vi "RT Driver VI.vi"(6 "Device Clock":string, 9 "Device Inputs FIFO":refnum<k33>, 10 "Device Outputs FIFO":refnum<k33>, 11 "Device Reference":T1 format="%.0x") -> ()   [LabVIEW 2020, in "Waveform Analog Output Engine.lvlib"]
uses:
  Waveform Analog Output Engine.lvlib
  <vilib>/NI VeriStand/Custom Device API/Custom Device Item Ref.ctl
  <vilib>/NI VeriStand/Custom Device API/Custom Device Channel Type.ctl
  <vilib>/Platform/TimedLoop/XDataNode/timing_clust.ctl
  <vilib>/Platform/TimedLoop/XDataNode/nitl_modes.ctl
  <vilib>/Platform/TimedLoop/XDataNode/wakeup.ctl
  <vilib>/NI VeriStand/Custom Device API/Message Response (String).ctl
  <vilib>/NI VeriStand/Custom Device API/Message Response (Byte Array).ctl
  <vilib>/DAQmx/write.llb/DAQmx Write (Analog 1D Wfm NChan NSamp).vi
  <vilib>/DAQmx/miscellaneous.llb/DAQmx Fill In Error Info.vi
  <vilib>/platform/TimedLoop/XDataNode/XDataNode.xnode
  <vilib>/NI VeriStand/Custom Device API/Custom Device API.lvlib
  <vilib>/NI VeriStand/Custom Device Tools/Custom Device Utility Library/Custom Device Utility Library.lvlib
  <resource>/objmgr/daqmx.rc
  <vilib>/Platform/TimedLoop/XDataNode/XDNodeRunTimeDep.lvlib
panel:
  out "Number of Overflow Occurred":i32
  out "Number of Underflow Occurred":i32
  out "L2 Output Buffer Usage":i32
  out "Actual Update Interval_Data Loop":dbl
  out "DAQ Error Code":i32
  out "Actual Update Interval_DAQ Loop":dbl
  out "Actual Sample Rate":dbl
  in  "Initialization Status Notifier":refnum<notifier>
  in  "Status Notifier":refnum<notifier>
  # "Custom Device Template\nv1.0"
  # "Use this template as a starting point for creating a custom device code module. The input controls shown here are specially named controls that the system will use to provide the device loop with data. The controls are not required for the device loop to run. For instance, if the device doesn't produce any output data, then you don't need the Device Outputs FIFO control. If you do use these controls, however, they need to have these exact names to be functional."
  # "status chs"
  # "The optional status notifier element is used to notify the RT engine of the last state of the custom device, and to indicate the device has completed execution. If this control is not used, a default No Error value is returned to the system when the device finishes execution.\n\nNote: This error state is not checked until the system shuts down. Use an output status channel to send more immediate status values to the system."
  # "This optional input can be used to send the VeriStand Engine the final status of the custom device initalization process. If this control exists on the custom device front panel, the VeriStand Engine will wait for a status update before starting up. If the custom device reports an error, that will abort the execution of the current configuration in the VeriStand Engine.\n\nThis control can be deleted if the custom device does not need to send the initialization status update."
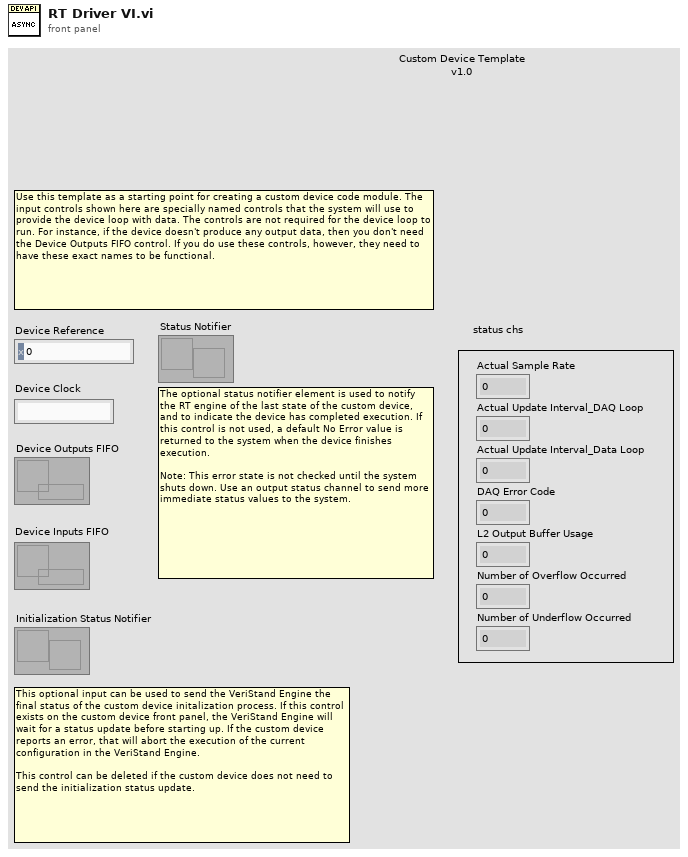
[diagram p1: front panel]
types:
  T1 = typedef "Custom Device API.lvlib/Custom Device Item Ref.ctl" = u64
  T2 = typedef "Custom Device API.lvlib/Custom Device Channel Type.ctl" = enum16{"Input", "Output"}
  T3 = typedef "Custom Device API.lvlib/Custom Device Engine Event Ref.ctl" = refnum<event-registration>
  T4 = typedef "Custom Device API.lvlib/Custom Device Timed Loop Priority.ctl" = enum32{"Low", "Medium", "High"}
  T5 = typedef "XDNodeRunTimeDep.lvlib/timing_clust.ctl" = cluster{"Expected End [f-1]":u64, "Actual End [f-1]":u64, "Finished Late? [f-1]":bool, "Expected End [i-1]":u64, "Actual End [i-1]":u64, "Finished Late? [i-1]":bool, "Expected Start [i]":u64, "Actual Start [i]":u64, "Expected Start [f]":u64, "Actual Start [f]":u64, "Source Name":string, "Structure Name":string, "Period":i64, "Deadline":i64, "Offset":i64, "Start":i64, "Priority":i32, "Timeout":i32, "Mode":T6, "Wakeup Reason":T7, "Error":errorcluster, "Source Type":string, "Secondary Source Type":string, "Global End Time":u64, "Global Start Time":u64, "Frame Duration":u64, "Iteration Duration":u64, "Assigned CPU":i32, "I/O Scan Engine Mode":u32}
  T6 = typedef "XDNodeRunTimeDep.lvlib/nitl_modes.ctl" = enum32{"No Change", "Process missed periods, maintain original phase", "Discard missed periods, maintain original phase", "Process missed periods, ignore original phase", "Discard missed periods, ignore original phase"}
  T7 = typedef "XDNodeRunTimeDep.lvlib/wakeup.ctl" = enum32{"Normal", "Aborted", "Asynchronous wakeup", "Timing source error", "Timed loop error", "Timeout"}
  T8 = typedef "Custom Device API.lvlib/Message Response (String).ctl" = cluster{"Response":string, "Error":errorcluster}
  T9 = typedef "Custom Device API.lvlib/Message Response (Byte Array).ctl" = cluster{"Response":u8[], "Error":errorcluster}
  T10 = typedef "Waveform Analog Output Engine.lvlib/DAQ Config Data.ctl" = cluster{"DAQPhysicalChannel(s)":string, "SampleRate":dbl, "MaxV":dbl, "MinV":dbl, "#Samples":dbl, "DataLoopInterval(ms)":u32, "StartDelay(ms)":dbl, "#L1OutputBuffers":i32, "#L2OutputBuffers":i32, "#Channels":i32, "ActualSampleRate(Hz)":dbl, "DAQTaskRef":refnum<k21>, "Latency":dbl}
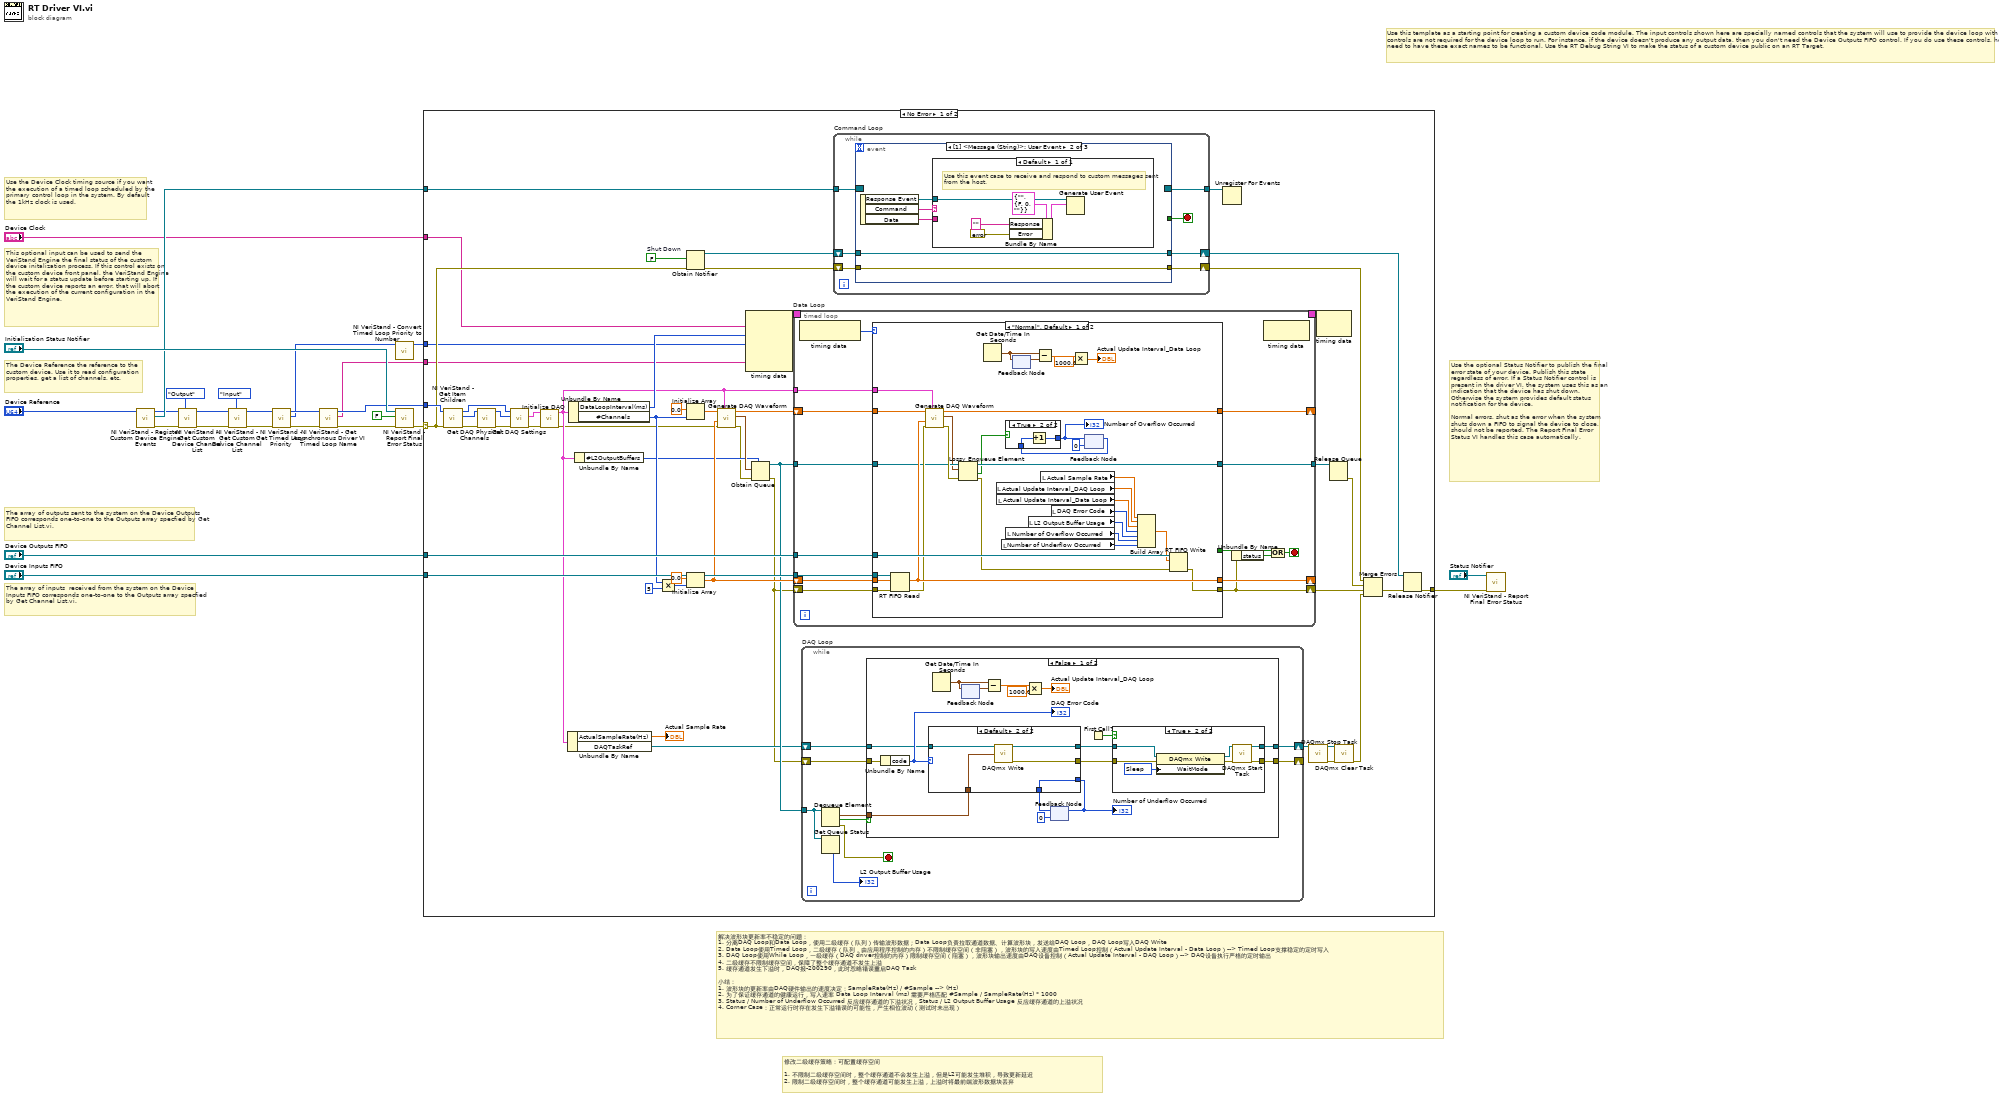
[diagram p0: block diagram]
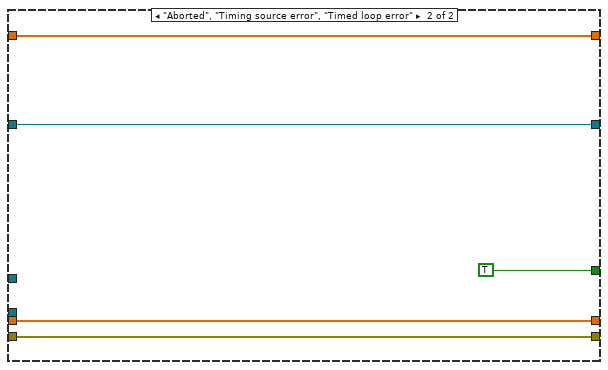
[diagram p3: hidden frame]
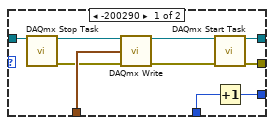
[diagram p4: hidden frame]
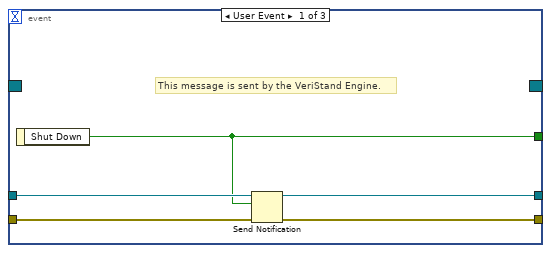
[diagram p7: hidden frame]
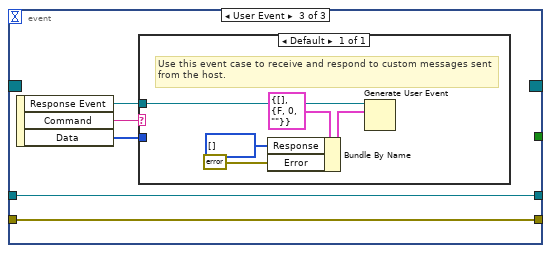
[diagram p8: hidden frame]
diagram:
  # "修改二级缓存策略：可配置缓存空间\n\n1. 不限制二级缓存空间时，整个缓存通道不会发生上溢，但是L2可能发生堆积，导致更新延迟\n2. 限制二级缓存空间时，整个缓存通道可能发生上溢，上溢时将最前端波形数据块丢弃"
  # "解决波形块更新率不稳定的问题：\n1. 分离DAQ Loop和Data Loop，使用二级缓存（队列）传输波形数据；Data Loop负责拉取通道数据、计算波形块，发送给DAQ Loop，DAQ Loop写入DAQ Write\n2. Data Loop使用Timed Loop，二级缓存（队列，由应用程序控制的内存）不限制缓存空间（非阻塞），波形块的写入速度由Timed Loop控制（Actual Update Interval - Data Loop）--> Timed Loop支撑稳定的定时写入\n3. DAQ Loop使用While Loop，一级缓存（DAQ driver控制的内存）限制缓存空间（阻塞），波形块输出速度由DAQ设备控制（Actual Update Interval - DAQ Loop）--> DAQ设备执行严格的定时输出\n4. 二级缓存不限制缓存空间，保障了整个缓存通道不发生上溢\n5. 缓存通道发生下溢时，DAQ报-200290，此时忽略错误重启DAQ Task\n\n小结：\n1. 波形块的更新率由DAQ硬件输出的速度决定：SampleRate(Hz) / #Sample --> (Hz)\n2. 为了保证缓存通道的健康运行，写入速率 Data Loop Interval (ms) 需要严格匹配 #Sample / SampleRate(Hz) * 1000\n3. Status / Number of Underflow Occurred 反应缓存通道的下溢状况，Status / L2 Output Buffer Usage 反应缓存通道的上溢状况\n4. Corner Case：正常运行时存在发生下溢错误的可能性，产生相位波动（测试时未出现）"
  # "This optional input can be used to send the VeriStand Engine the final status of the custom device initalization process. If this control exists on the custom device front panel, the VeriStand Engine will wait for a status update before starting up. If the custom device reports an error, that will abort the execution of the current configuration in the VeriStand Engine."
  # "The array of inputs  received from the system on the Device Inputs FIFO corresponds one-to-one to the Outputs array specfied by Get Channel List.vi."
  # "Use the optional Status Notifier to publish the final error state of your device. Publish this state regardless of error. If a Status Notifier control is present in the driver VI, the system uses this as an indication that the device has shut down. Otherwise the system provides default status notification for the device.\n\nNormal errors, shut as the error when the system shuts down a FIFO to signal the device to close, should not be reported. The Report Final Error Status VI handles this case automatically."
  # "The array of outputs sent to the system on the Device Outputs FIFO corresponds one-to-one to the Outputs array specfied by Get Channel List.vi."
  # "The Device Reference the reference to the custom device. Use it to read configuration properties, get a list of channels, etc."
  # "Use the Device Clock timing source if you want the execution of a timed loop scheduled by the primary control loop in the system. By default the 1kHz clock is used."
  # "Use this template as a starting point for creating a custom device code module. The input controls shown here are specially named controls that the system will use to provide the device loop with data. The controls are not required for the device loop to run. For instance, if the device doesn't produce any output data, then you don't need the Device Outputs FIFO control. If you do use these controls, however, they need to have these exact names to be functional. Use the RT Debug String VI to make the status of a custom device public on an RT Target."
  n1 = call <vilib>:"NI VeriStand - Register Custom Device Engine Events.vi"("Device Ref in"="Device Reference") -> ("error out"=w25:errorcluster, "Custom Device Engine Event Ref"=w16:T3, "Device Ref out"=w14:T1)  [unwired: 8 in]
  n2 = call <vilib>:"NI VeriStand - Get Custom Device Channel List.vi"("Channel Type"=Custom_Device_Channel_Type."Output", "error in (no error)"=w25, "Device Ref in"=w14) -> ("error out"=w19:errorcluster, "Device Ref out"=w20:T1)  [unwired: 7 out]
  n3 = call <vilib>:"NI VeriStand - Get Custom Device Channel List.vi"("Channel Type"=Custom_Device_Channel_Type."Input", "error in (no error)"=w19, "Device Ref in"=w20) -> ("error out"=w3:errorcluster, "Device Ref out"=w12:T1)  [unwired: 7 out]
  n4 = call <vilib>:"NI VeriStand - Get Timed Loop Priority.vi"("error in (no error)"=w3, "Device Ref in"=w12) -> ("error out"=w2:errorcluster, "Priority"=w7:T4, "Device Ref out"=w9:T1)  [unwired: 7 in]
  n5 = call <vilib>:"NI VeriStand - Get Asynchronous Driver VI Timed Loop Name.vi"("error in (no error)"=w2, "Device Ref in"=w9) -> ("error out"=w1:errorcluster, "Device Timed Loop Name"=w4:string, "Device Ref out"=w5:T1)  [unwired: 7 in]
  n6 = call <vilib>:"NI VeriStand - Convert Timed Loop Priority to Number.vi"("Priority"=w7) -> ("Numeric Priority"=w6:i32)  [unwired: 10 in]
  n7 = call <vilib>:"NI VeriStand - Report Final Error Status.vi"("error in (no error)"=w1, "Filter FIFO & Shutdown Errors (T)"=FALSE ("Filter FIFO Errors (T)"), "Status Notifier"="Initialization Status Notifier") -> ("error out"=w10:errorcluster)  [unwired: 8 out]
  n8 = case shown="No Error" w10 {
    selector: w10 -> [w53 w225]
    tunnel: "Device Outputs FIFO" -> [w74 _]
    tunnel: "Device Inputs FIFO" -> [w73 _]
    tunnel: w16 -> [w71 _]
    tunnel: [w69 w225] -> w15
    tunnel: w5 -> [w62 _]
    tunnel: "Device Clock" -> [w37 _]
    tunnel: w6 -> [w36 _]
    tunnel: w4 -> [w35 _]
    frame No Error {
      w70 = FALSE  # Shut Down
      n9 = call <vilib>:"NI VeriStand - Get Item Children.vi"("error in (no error)"=w53, "Item Ref in"=w62) -> ("error out"=w64:errorcluster, "Child Refs"=w59:T1[], "Item Ref out"=w60:T1)  [unwired: 6 in, 1 out]
      n10 = call "Get DAQ Physical Channels.vi"("error in (no error)"=w64, "DAQ Channel Section Refs"=w59) -> ("error out"=w63:errorcluster, "Physical Channels"=w61:i32[])  [unwired: 8 in]
      n11 = call "Get DAQ Settings.vi"("error in (no error)"=w63, "Physical Chan Array"=w61, "Device Ref in"=w60) -> ("error out"=w52:errorcluster, "DAQ Config Data"=w51:T10)  [unwired: 6 in, 1 out]
      n12 = call "Initialize DAQ.vi"("error in (no error)"=w52, "DAQ Config Data In"=w51) -> ("error out"=w27:errorcluster, "DAQ Config Data Out"=w28:T10)  [unwired: 8 in]
      n13 = Unbundle By Name(w28) -> ("ActualSampleRate(Hz)"=→"Actual Sample Rate":dbl, "DAQTaskRef"=w43:refnum<k21>)
      n14 = Unbundle By Name(w28) -> ("DataLoopInterval(ms)"=w38:u32, "#Channels"=w55:i32)
      n15 = Unbundle By Name(w28) -> ("#L2OutputBuffers"=w29:i32)
      n16 = Multiply(x=w55, y=5) -> (x*y=w57:i32)
      n17 = Obtain Notifier(notification data type=w70, error in (no error)=w53) -> (notifier out=w67:refnum<notifier>, error out=w75:errorcluster)  [unwired: 2 in, 1 out]
      n18 = Initialize Array(0.0 ("element"), w55) -> (w50:dbl[])
      n19 = Initialize Array(0.0 ("element"), w57) -> (w48:dbl[])
      n20 = call "Generate DAQ Waveform.vi"("DAQ Config Data"=w28, "error in (no error)"=w27, "Channel Data"=w48, "Phase Array In"=w50) -> ("error out"=w26:errorcluster, "Waveform Array"=w41:waveform(dbl)[], "Phase Array Out out"=w49:dbl[])  [unwired: 5 in]
      n21 = node-c288(w37, w38, w36, w35) -> (w40:T5)  [unwired: 1 in]
      n22 = Obtain Queue(max queue size (-1, unlimited)=w29, element data type=w41, error in (no error)=w26) -> (queue out=w46:refnum<queue>, error out=w42:errorcluster)  [unwired: 2 in, 1 out]
      n23 = timed-loop "Data Loop" {
        shift-right: [w88] -> _
        shift-left: w48 -> [w89]
        shift-right: [w85] -> w44
        shift-left: w42 -> [w90]
        tunnel: w74 -> [w87]
        tunnel: w73 -> [w86]
        shift-right: [w80] -> _
        shift-left: w49 -> [w81]
        tunnel: w28 -> [w79]
        tunnel: w46 -> [w78]
        tunnel: [w77] -> w45
        timing: w40 -> [_]
        timing-out: [_] -> w39
        stop <- w82 stop-if-true
        n24 = node-c288() -> (w76:T7)  [unwired: 1 in]
        n25 = case shown="\"Normal\", Default" w76 {
          tunnel: w90 -> [w117 w132]
          tunnel: w89 -> [w121 w133]
          tunnel: [w120 w133] -> w88
          tunnel: w87 -> [w125 _]
          tunnel: w86 -> [w124 _]
          tunnel: [w119 w132] -> w85
          tunnel: [_ TRUE] -> w83
          tunnel: w81 -> [w122 w130]
          tunnel: [w123 w130] -> w80
          tunnel: w79 -> [w118 _]
          tunnel: w78 -> [w114 w129]
          tunnel: [w99 w129] -> w77
          frame "Normal", Default {
            n26 = RT FIFO Read(0:w124, 1:w121, 3:w117) -> (9:w120:dbl[], 11:w116:errorcluster)  [unwired: 4 out]
            n27 = call "Generate DAQ Waveform.vi"("DAQ Config Data"=w118, "error in (no error)"=w116, "Channel Data"=w120, "Phase Array In"=w122) -> ("error out"=w115:errorcluster, "Waveform Array"=w112:waveform(dbl)[], "Phase Array Out out"=w123:dbl[])  [unwired: 5 in]
            n28 = Lossy Enqueue Element(queue=w114, element=w112, error in (no error)=w115) -> (queue out=w99:refnum<queue>, overflow?=w98:bool, error out=w113:errorcluster)  [unwired: 1 out]
            n29 = Get Date/Time In Seconds() -> (seconds since 1Jan1904=w108:timestamp)
            n30 = local read "Actual Update Interval_DAQ Loop"() -> (w102:dbl)
            n31 = local read "Actual Update Interval_Data Loop"() -> (w103:dbl)
            n32 = local read "Number of Underflow Occurred"() -> (w106:i32)
            n33 = local read "Number of Overflow Occurred"() -> (w94:i32)
            n34 = feedback #1() -> (w109:timestamp)  [unwired: 1 in]
            n35 = feedback-in #1(w108) -> ()
            n36 = local read "L2 Output Buffer Usage"() -> (w100:i32)
            n37 = Subtract(x=w108, y=w109) -> (x-y=w110:dbl)
            n38 = local read "Actual Sample Rate"() -> (w105:dbl)
            n39 = local read "DAQ Error Code"() -> (w104:i32)
            n40 = Multiply(x=w110, y=1000.0) -> (x*y=→"Actual Update Interval_Data Loop":dbl)
            n41 = feedback #2(0) -> (w96:i32)
            n42 = case shown="True" w98 {
              tunnel: w96 -> [w126 w128]
              tunnel: [w126 w127] -> w95
              frame False {
              }
              frame True {
                n43 = Increment(x=w128) -> (x+1=w127:i32)
              }
            }
            "Number of Overflow Occurred" <- w95
            n44 = feedback-in #2(w95) -> ()
            n45 = Build Array(w105, w102, w103, w104, w100, w94, w106) -> (w101:dbl[])
            n46 = RT FIFO Write(0:w125, 1:w101, 3:w113) -> (11:w119:errorcluster)  [unwired: 1 in, 4 out]
          }
          frame "Aborted", "Timing source error", "Timed loop error" {
          }
        }
        n47 = Unbundle By Name(w85) -> ("status"=w84:bool)
        n48 = node-c288() -> ()  [unwired: 1 in, 1 out]
        n49 = Compound Arithmetic op=OR(w83, w84) -> (w82:bool)
      }
      n50 = while "DAQ Loop" {
        shift-right: [w149] -> w47
        shift-left: w43 -> [w148]
        tunnel: w46 -> [w141]
        shift-right: [w145] -> _
        shift-left: w42 -> [w144]
        stop <- w143 stop-if-true
        n51 = Dequeue Element(queue=w141) -> (element=w146:waveform(dbl)[], timed out?=w147:bool, error out=w143:errorcluster)  [unwired: 2 in, 1 out]
        n52 = Get Queue Status(queue=w141) -> (# elements in queue=→"L2 Output Buffer Usage":i32)  [unwired: 2 in, 7 out]
        n53 = case shown="False" w147 {
          tunnel: [w165 w192] -> w149
          tunnel: w148 -> [w157 w192]
          tunnel: w146 -> [w156 _]
          tunnel: [w160 w191] -> w145
          tunnel: w144 -> [w159 w191]
          frame False {
            n54 = Unbundle By Name(w159) -> ("code"=w158:i32)
            "DAQ Error Code" <- w158
            n55 = Get Date/Time In Seconds() -> (seconds since 1Jan1904=w161:timestamp)
            n56 = feedback #3() -> (w162:timestamp)  [unwired: 1 in]
            n57 = feedback-in #3(w161) -> ()
            n58 = Subtract(x=w161, y=w162) -> (x-y=w163:dbl)
            n59 = Multiply(x=w163, y=1000.0) -> (x*y=→"Actual Update Interval_DAQ Loop":dbl)
            n60 = feedback #4(0) -> (w152:i32)
            n61 = case shown="Default" w158 {
              tunnel: [w176 w179] -> w154
              tunnel: w157 -> [w175 w180]
              tunnel: w156 -> [w174 w181]
              tunnel: [w169 w178] -> w155
              tunnel: [w167 w177] -> w151
              tunnel: w152 -> [w168 w177]
              frame -200290 {
                n62 = call <vilib>:"DAQmx Stop Task.vi"("task/channels in"=w175) -> ("task out"=w173:refnum<k21>, "error out"=w172:errorcluster)  [unwired: 13 in]
                n63 = call-poly <vilib>:"DAQmx Write.vi"("task/channels in"=w173, "data"=w174, "error in"=w172) -> ("task out"=w170:refnum<k21>, "error out"=w171:errorcluster)  [unwired: 10 in, 1 out]
                n64 = call <vilib>:"DAQmx Start Task.vi"("task/channels in"=w170, "error in"=w171) -> ("task out"=w169:refnum<k21>, "error out"=w176:errorcluster)  [unwired: 12 in]
                n65 = Increment(x=w168) -> (x+1=w167:i32)
              }
              frame Default {
                n66 = call-poly <vilib>:"DAQmx Write.vi"("task/channels in"=w180, "data"=w181) -> ("task out"=w178:refnum<k21>, "error out"=w179:errorcluster)  [unwired: 11 in, 1 out]
              }
            }
            "Number of Underflow Occurred" <- w151
            n67 = feedback-in #4(w151) -> ()
            n68 = First Call?() -> (First Call?: T/F=w166:bool)
            n69 = case shown="True" w166 {
              tunnel: w155 -> [w183 w187]
              tunnel: [w183 w186] -> w165
              tunnel: w154 -> [w182 w185]
              tunnel: [w182 w184] -> w160
              frame False {
              }
              frame True {
                w188 = 12547 items=["Poll"=12524, "Yield"=12525, "Sleep"=12547] ("WaitMode")
                n70 = property class="DAQmx Write"(reference=w187, error in=w185, "WaitMode"=w188) -> (reference out=w190:refnum<k21>, error out=w189:errorcluster)
                n71 = call <vilib>:"DAQmx Start Task.vi"("task/channels in"=w190, "error in"=w189) -> ("task out"=w186:refnum<k21>, "error out"=w184:errorcluster)  [unwired: 12 in]
              }
            }
          }
          frame True {
          }
        }
      }
      n72 = while "Command Loop" {
        tunnel: w71 -> [w199]
        tunnel: [w198] -> w68
        shift-right: [w195] -> w66
        shift-left: w67 -> [w196]
        shift-right: [w193] -> w31
        shift-left: w75 -> [w194]
        stop <- w197 stop-if-true
        n73 = event shown="[1] <Message (String)>: User Event" {
          selector: w199 -> [_ _ _]
          dyn-events: [_ _ _] -> w198
          timeout: _ -> [_ _ _]
          tunnel: [w202 _ _] -> w197
          tunnel: w196 -> [w203 w207 w217]
          tunnel: [w204 w207 w217] -> w195
          tunnel: w194 -> [w201 w205 w215]
          tunnel: [w200 w205 w215] -> w193
          event User Event {
            # "This message is sent by the VeriStand Engine."
            n74 = event-data() -> ("Shut Down"=w202:bool)  [unwired: 1 in]
            n75 = Send Notification(notification=w202, notifier=w203, error in (no error)=w201) -> (notifier out=w204:refnum<notifier>, error out=w200:errorcluster)
          }
          event User Event {
            n76 = event-data() -> ("Response Event"=w206:refnum<user-event>, "Command"=w209:string, "Data"=w208:string)  [unwired: 1 in]
            n77 = case shown="Default" w209 {
              tunnel: w208 -> [_]
              tunnel: w206 -> [w214]
              frame Default {
                # "Use this event case to receive and respond to custom messages sent from the host."
                n78 = Bundle By Name(cluster=T8 {"Response"="", "Error"={"status"=FALSE, "code"=0, "source"=""}} ("event data"), "Response"="", "Error"=errorcluster {"status"=FALSE, "code"=0, "source"=""}) -> (w212:T8)
                n79 = Generate User Event(user event=w214, event data cluster=w212) -> ()  [unwired: 2 in, 2 out]
              }
            }
          }
          event User Event {
            n80 = event-data() -> ("Response Event"=w216:refnum<user-event>, "Command"=w219:string, "Data"=w218:u8[])  [unwired: 1 in]
            n81 = case shown="Default" w219 {
              tunnel: w218 -> [_]
              tunnel: w216 -> [w224]
              frame Default {
                # "Use this event case to receive and respond to custom messages sent from the host."
                n82 = Bundle By Name(cluster=T9 {"Response"=[], "Error"={"status"=FALSE, "code"=0, "source"=""}} ("event data"), "Response"=u8[] [], "Error"=errorcluster {"status"=FALSE, "code"=0, "source"=""}) -> (w221:T9)
                n83 = Generate User Event(user event=w224, event data cluster=w221) -> ()  [unwired: 2 in, 2 out]
              }
            }
          }
        }
      }
      n84 = Unregister For Events(event registration refnum=w68) -> ()  [unwired: 1 in, 1 out]
      n85 = call <vilib>:"DAQmx Stop Task.vi"("task/channels in"=w47) -> ("task out"=w54:refnum<k21>, "error out"=w33:errorcluster)  [unwired: 13 in]
      n86 = node-c288(w39) -> ()  [unwired: 1 out]
      n87 = Release Queue(queue=w45) -> (error out=w30:errorcluster)  [unwired: 2 in, 2 out]
      n88 = call <vilib>:"DAQmx Clear Task.vi"("task in"=w54, "error in"=w33) -> ("error out"=w32:errorcluster)  [unwired: 13 in]
      n89 = Merge Errors(w31, w30, w44, w32) -> (w65:errorcluster)
      n90 = Release Notifier(notifier=w66, error in (no error)=w65) -> (error out=w69:errorcluster)  [unwired: 1 in, 2 out]
    }
    frame Error {
    }
  }
  n91 = call <vilib>:"NI VeriStand - Report Final Error Status.vi"("error in (no error)"=w15, "Status Notifier"="Status Notifier") -> ()  [unwired: 1 in, 9 out]
